vi "Keithley2450 Piano.vi"() -> ()   [LabVIEW 2020]
uses:
  <instrlib>/Keithley 2450/Keithley 2450.lvlib
panel:
  in  "?":bool
  in  "VISA resource name":refnum<visa-resource-name>
  in  "?":bool
  in  "?":bool
  in  "?":bool
  in  "?":bool
  in  "?":bool
  in  "?":bool
  in  "?":bool
  in  "?":bool
  in  "?":bool
  in  "?":bool
  in  "?":bool
  in  "?":bool
  in  "?":bool
  in  "?":bool
  in  "?":bool
  in  "?":bool
  in  "?":bool
  in  "?":bool
  in  "?":bool
  in  "?":bool
  in  "?":bool
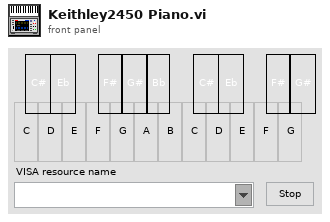
[diagram p1: front panel]
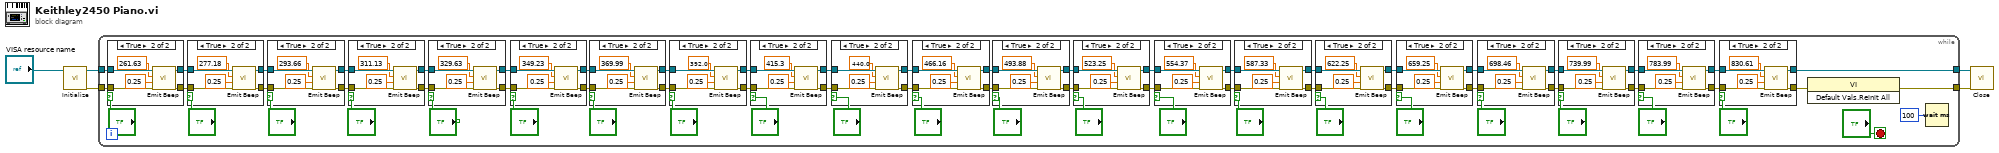
[diagram p0: block diagram]
diagram:
  n1 = call <instrlib>:"Initialize.vi"("VISA resource name"="VISA resource name") -> ("error out"=w3:errorcluster, "VISA resource name out"=w4:refnum<visa-resource-name>)  [unwired: 9 in]
  n2 = while {
    tunnel: w4 -> [w72]
    tunnel: w3 -> [w71]
    tunnel: [w20] -> w1
    tunnel: [w7] -> w2
    stop <- "?" stop-if-true
    n3 = case shown="True" "?" {
      tunnel: w72 -> [w235 w241]
      tunnel: w71 -> [w234 w240]
      tunnel: [w235 w237] -> w68
      tunnel: [w234 w236] -> w67
      frame False {
      }
      frame True {
        n4 = call <instrlib>:"Emit Beep.vi"("error in (no error)"=w240, "Beep Duration (.25 s)"=0.25, "Beep Frequency (300)"=261.63, "VISA resource name"=w241) -> ("error out"=w236:errorcluster, "VISA resource name out"=w237:refnum<visa-resource-name>)  [unwired: 6 in]
      }
    }
    n5 = case shown="True" "?" {
      tunnel: w68 -> [w227 w233]
      tunnel: w67 -> [w226 w232]
      tunnel: [w227 w229] -> w66
      tunnel: [w226 w228] -> w65
      frame False {
      }
      frame True {
        n6 = call <instrlib>:"Emit Beep.vi"("error in (no error)"=w232, "Beep Duration (.25 s)"=0.25, "Beep Frequency (300)"=277.18, "VISA resource name"=w233) -> ("error out"=w228:errorcluster, "VISA resource name out"=w229:refnum<visa-resource-name>)  [unwired: 6 in]
      }
    }
    n7 = case shown="True" "?" {
      tunnel: w66 -> [w219 w225]
      tunnel: w65 -> [w218 w224]
      tunnel: [w219 w221] -> w59
      tunnel: [w218 w220] -> w58
      frame False {
      }
      frame True {
        n8 = call <instrlib>:"Emit Beep.vi"("error in (no error)"=w224, "Beep Duration (.25 s)"=0.25, "Beep Frequency (300)"=293.66, "VISA resource name"=w225) -> ("error out"=w220:errorcluster, "VISA resource name out"=w221:refnum<visa-resource-name>)  [unwired: 6 in]
      }
    }
    n9 = case shown="True" "?" {
      tunnel: w59 -> [w211 w217]
      tunnel: w58 -> [w210 w216]
      tunnel: [w211 w213] -> w57
      tunnel: [w210 w212] -> w56
      frame False {
      }
      frame True {
        n10 = call <instrlib>:"Emit Beep.vi"("error in (no error)"=w216, "Beep Duration (.25 s)"=0.25, "Beep Frequency (300)"=311.13, "VISA resource name"=w217) -> ("error out"=w212:errorcluster, "VISA resource name out"=w213:refnum<visa-resource-name>)  [unwired: 6 in]
      }
    }
    n11 = case shown="True" "?" {
      tunnel: w57 -> [w203 w209]
      tunnel: w56 -> [w202 w208]
      tunnel: [w203 w205] -> w55
      tunnel: [w202 w204] -> w54
      frame False {
      }
      frame True {
        n12 = call <instrlib>:"Emit Beep.vi"("error in (no error)"=w208, "Beep Duration (.25 s)"=0.25, "Beep Frequency (300)"=329.63, "VISA resource name"=w209) -> ("error out"=w204:errorcluster, "VISA resource name out"=w205:refnum<visa-resource-name>)  [unwired: 6 in]
      }
    }
    n13 = case shown="True" "?" {
      tunnel: w55 -> [w195 w201]
      tunnel: w54 -> [w194 w200]
      tunnel: [w195 w197] -> w53
      tunnel: [w194 w196] -> w52
      frame False {
      }
      frame True {
        n14 = call <instrlib>:"Emit Beep.vi"("error in (no error)"=w200, "Beep Duration (.25 s)"=0.25, "Beep Frequency (300)"=349.23, "VISA resource name"=w201) -> ("error out"=w196:errorcluster, "VISA resource name out"=w197:refnum<visa-resource-name>)  [unwired: 6 in]
      }
    }
    n15 = case shown="True" "?" {
      tunnel: w53 -> [w187 w193]
      tunnel: w52 -> [w186 w192]
      tunnel: [w187 w189] -> w51
      tunnel: [w186 w188] -> w50
      frame False {
      }
      frame True {
        n16 = call <instrlib>:"Emit Beep.vi"("error in (no error)"=w192, "Beep Duration (.25 s)"=0.25, "Beep Frequency (300)"=369.99, "VISA resource name"=w193) -> ("error out"=w188:errorcluster, "VISA resource name out"=w189:refnum<visa-resource-name>)  [unwired: 6 in]
      }
    }
    n17 = case shown="True" "?" {
      tunnel: w51 -> [w179 w185]
      tunnel: w50 -> [w178 w184]
      tunnel: [w179 w181] -> w49
      tunnel: [w178 w180] -> w48
      frame False {
      }
      frame True {
        n18 = call <instrlib>:"Emit Beep.vi"("error in (no error)"=w184, "Beep Duration (.25 s)"=0.25, "Beep Frequency (300)"=392.0, "VISA resource name"=w185) -> ("error out"=w180:errorcluster, "VISA resource name out"=w181:refnum<visa-resource-name>)  [unwired: 6 in]
      }
    }
    n19 = case shown="True" "?" {
      tunnel: w49 -> [w171 w177]
      tunnel: w48 -> [w170 w176]
      tunnel: [w171 w173] -> w44
      tunnel: [w170 w172] -> w45
      frame False {
      }
      frame True {
        n20 = call <instrlib>:"Emit Beep.vi"("error in (no error)"=w176, "Beep Duration (.25 s)"=0.25, "Beep Frequency (300)"=415.3, "VISA resource name"=w177) -> ("error out"=w172:errorcluster, "VISA resource name out"=w173:refnum<visa-resource-name>)  [unwired: 6 in]
      }
    }
    n21 = case shown="True" "?" {
      tunnel: w44 -> [w163 w169]
      tunnel: w45 -> [w162 w168]
      tunnel: [w163 w165] -> w43
      tunnel: [w162 w164] -> w42
      frame False {
      }
      frame True {
        n22 = call <instrlib>:"Emit Beep.vi"("error in (no error)"=w168, "Beep Duration (.25 s)"=0.25, "Beep Frequency (300)"=440.0, "VISA resource name"=w169) -> ("error out"=w164:errorcluster, "VISA resource name out"=w165:refnum<visa-resource-name>)  [unwired: 6 in]
      }
    }
    n23 = case shown="True" "?" {
      tunnel: w43 -> [w155 w161]
      tunnel: w42 -> [w154 w160]
      tunnel: [w155 w157] -> w40
      tunnel: [w154 w156] -> w39
      frame False {
      }
      frame True {
        n24 = call <instrlib>:"Emit Beep.vi"("error in (no error)"=w160, "Beep Duration (.25 s)"=0.25, "Beep Frequency (300)"=466.16, "VISA resource name"=w161) -> ("error out"=w156:errorcluster, "VISA resource name out"=w157:refnum<visa-resource-name>)  [unwired: 6 in]
      }
    }
    n25 = case shown="True" "?" {
      tunnel: w40 -> [w147 w153]
      tunnel: w39 -> [w146 w152]
      tunnel: [w147 w149] -> w37
      tunnel: [w146 w148] -> w38
      frame False {
      }
      frame True {
        n26 = call <instrlib>:"Emit Beep.vi"("error in (no error)"=w152, "Beep Duration (.25 s)"=0.25, "Beep Frequency (300)"=493.88, "VISA resource name"=w153) -> ("error out"=w148:errorcluster, "VISA resource name out"=w149:refnum<visa-resource-name>)  [unwired: 6 in]
      }
    }
    n27 = case shown="True" "?" {
      tunnel: w37 -> [w139 w145]
      tunnel: w38 -> [w138 w144]
      tunnel: [w139 w141] -> w36
      tunnel: [w138 w140] -> w35
      frame False {
      }
      frame True {
        n28 = call <instrlib>:"Emit Beep.vi"("error in (no error)"=w144, "Beep Duration (.25 s)"=0.25, "Beep Frequency (300)"=523.25, "VISA resource name"=w145) -> ("error out"=w140:errorcluster, "VISA resource name out"=w141:refnum<visa-resource-name>)  [unwired: 6 in]
      }
    }
    n29 = case shown="True" "?" {
      tunnel: w36 -> [w131 w137]
      tunnel: w35 -> [w130 w136]
      tunnel: [w131 w133] -> w34
      tunnel: [w130 w132] -> w33
      frame False {
      }
      frame True {
        n30 = call <instrlib>:"Emit Beep.vi"("error in (no error)"=w136, "Beep Duration (.25 s)"=0.25, "Beep Frequency (300)"=554.37, "VISA resource name"=w137) -> ("error out"=w132:errorcluster, "VISA resource name out"=w133:refnum<visa-resource-name>)  [unwired: 6 in]
      }
    }
    n31 = case shown="True" "?" {
      tunnel: w34 -> [w123 w129]
      tunnel: w33 -> [w122 w128]
      tunnel: [w123 w125] -> w32
      tunnel: [w122 w124] -> w31
      frame False {
      }
      frame True {
        n32 = call <instrlib>:"Emit Beep.vi"("error in (no error)"=w128, "Beep Duration (.25 s)"=0.25, "Beep Frequency (300)"=587.33, "VISA resource name"=w129) -> ("error out"=w124:errorcluster, "VISA resource name out"=w125:refnum<visa-resource-name>)  [unwired: 6 in]
      }
    }
    n33 = case shown="True" "?" {
      tunnel: w32 -> [w115 w121]
      tunnel: w31 -> [w114 w120]
      tunnel: [w115 w117] -> w30
      tunnel: [w114 w116] -> w29
      frame False {
      }
      frame True {
        n34 = call <instrlib>:"Emit Beep.vi"("error in (no error)"=w120, "Beep Duration (.25 s)"=0.25, "Beep Frequency (300)"=622.25, "VISA resource name"=w121) -> ("error out"=w116:errorcluster, "VISA resource name out"=w117:refnum<visa-resource-name>)  [unwired: 6 in]
      }
    }
    n35 = case shown="True" "?" {
      tunnel: w30 -> [w107 w113]
      tunnel: w29 -> [w106 w112]
      tunnel: [w107 w109] -> w28
      tunnel: [w106 w108] -> w27
      frame False {
      }
      frame True {
        n36 = call <instrlib>:"Emit Beep.vi"("error in (no error)"=w112, "Beep Duration (.25 s)"=0.25, "Beep Frequency (300)"=659.25, "VISA resource name"=w113) -> ("error out"=w108:errorcluster, "VISA resource name out"=w109:refnum<visa-resource-name>)  [unwired: 6 in]
      }
    }
    n37 = case shown="True" "?" {
      tunnel: w28 -> [w99 w105]
      tunnel: w27 -> [w98 w104]
      tunnel: [w99 w101] -> w26
      tunnel: [w98 w100] -> w25
      frame False {
      }
      frame True {
        n38 = call <instrlib>:"Emit Beep.vi"("error in (no error)"=w104, "Beep Duration (.25 s)"=0.25, "Beep Frequency (300)"=698.46, "VISA resource name"=w105) -> ("error out"=w100:errorcluster, "VISA resource name out"=w101:refnum<visa-resource-name>)  [unwired: 6 in]
      }
    }
    n39 = case shown="True" "?" {
      tunnel: w26 -> [w91 w97]
      tunnel: w25 -> [w90 w96]
      tunnel: [w91 w93] -> w24
      tunnel: [w90 w92] -> w23
      frame False {
      }
      frame True {
        n40 = call <instrlib>:"Emit Beep.vi"("error in (no error)"=w96, "Beep Duration (.25 s)"=0.25, "Beep Frequency (300)"=739.99, "VISA resource name"=w97) -> ("error out"=w92:errorcluster, "VISA resource name out"=w93:refnum<visa-resource-name>)  [unwired: 6 in]
      }
    }
    n41 = case shown="True" "?" {
      tunnel: w24 -> [w83 w89]
      tunnel: w23 -> [w82 w88]
      tunnel: [w83 w85] -> w22
      tunnel: [w82 w84] -> w21
      frame False {
      }
      frame True {
        n42 = call <instrlib>:"Emit Beep.vi"("error in (no error)"=w88, "Beep Duration (.25 s)"=0.25, "Beep Frequency (300)"=783.99, "VISA resource name"=w89) -> ("error out"=w84:errorcluster, "VISA resource name out"=w85:refnum<visa-resource-name>)  [unwired: 6 in]
      }
    }
    n43 = case shown="True" "?" {
      tunnel: w22 -> [w75 w81]
      tunnel: w21 -> [w74 w80]
      tunnel: [w75 w77] -> w20
      tunnel: [w74 w76] -> w8
      frame False {
      }
      frame True {
        n44 = call <instrlib>:"Emit Beep.vi"("error in (no error)"=w80, "Beep Duration (.25 s)"=0.25, "Beep Frequency (300)"=830.61, "VISA resource name"=w81) -> ("error out"=w76:errorcluster, "VISA resource name out"=w77:refnum<visa-resource-name>)  [unwired: 6 in]
      }
    }
    n45 = invoke class="VI" method="Default Vals.Reinit All"(error in=w8) -> (error out=w7:errorcluster)  [unwired: 2 in, 2 out]
    n46 = Wait (ms)(milliseconds to wait=u32 100) -> ()  [unwired: 1 out]
  }
  n47 = call <instrlib>:"Close.vi"("error in (no error)"=w2, "VISA resource name"=w1) -> ()  [unwired: 9 in, 1 out]
